vi "Handle pending Requests.vi"(8 "error in (no error)":errorcluster, 11 "IP Connection in":refnum<class "IP Connection.lvclass">) -> (0 "error out":errorcluster, 3 "IP Connection out":refnum<class "IP Connection.lvclass">)   [LabVIEW 2011, in "Tinkerforge.lvlib" / "IP Connection.lvclass"]
doc: "This VI handles pending requests and sends an timeout answer if necessary."
uses:
  IP Connection.lvclass
  IP Connection.lvclass/IP Connection.ctl
  Type Definitions/Request Identifier.ctl
  Type Definitions/Errors.ctl
  Type Definitions/Request Type.ctl
  Type Definitions/Answer.ctl
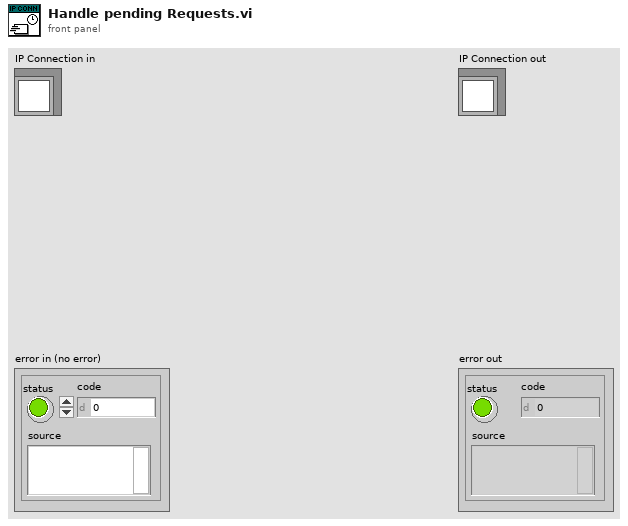
[diagram p1: front panel]
types:
  T1 = typedef "Tinkerforge.lvlib/IP Connection.lvclass/Request Identifier.ctl" = cluster{"Stack ID":u8, "Function ID":u8, "Request GUID":string, "Remaining Timeout":i32}
  T2 = typedef "Tinkerforge.lvlib/IP Connection.lvclass/Errors.ctl" = enum16{"Timeout", "Device type incorrect", "Device already added", "Device not existing"}
  T3 = typedef "Tinkerforge.lvlib/IP Connection.lvclass/Request Type.ctl" = enum8{"Invalid", "Write"}
  T4 = typedef "Tinkerforge.lvlib/IP Connection.lvclass/Answer.ctl" = cluster{"Request GUID":string, "Request Type":T3, "Sucessful":bool, "Data":variant, "Error":errorcluster}
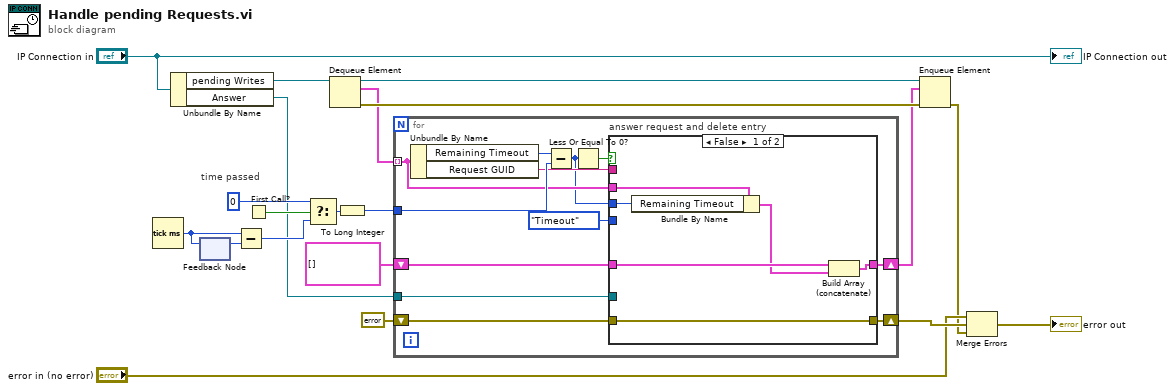
[diagram p0: block diagram]
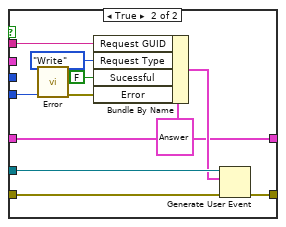
[diagram p2: hidden frame]
diagram:
  # "time passed"
  n1 = Tick Count (ms)() -> (millisecond timer value=w14:u32)
  n2 = Unbundle By Name("IP Connection in") -> ("pending Writes"=w18:refnum<queue>, "Answer"=w7:refnum<user-event>)
  n3 = feedback #1() -> (w15:u32)  [unwired: 1 in]
  n4 = feedback-in #1(w14) -> ()
  n5 = Subtract(x=w14, y=w15) -> (x-y=w13:u32)
  n6 = First Call?() -> (First Call?: T/F=w12:bool)
  n7 = Select(t=u32 0, s=w12, f=w13) -> (s? t:f=w10:u32)
  n8 = Dequeue Element(queue=w18) -> (queue out=w17:refnum<queue>, element=w8:T1[], error out=w16:errorcluster)  [unwired: 2 in, 1 out]
  n9 = To Long Integer(number=w10) -> (32bit integer=w9:i32)
  n10 = for {
    tunnel: w8 -> [w24] mode=indexing
    tunnel: w9 -> [w31]
    shift-right: [w23] -> w5
    shift-left: T1[] [] -> [w28]
    shift-right: [w27] -> w4
    shift-left: errorcluster {"status"=FALSE, "code"=0, "source"=""} ("error out") -> [w30]
    tunnel: w7 -> [w25]
    n11 = Unbundle By Name(w24) -> ("Remaining Timeout"=w32:i32, "Request GUID"=w26:string)
    n12 = Subtract(x=w32, y=w31) -> (x-y=w21:i32)
    n13 = Less Or Equal To 0?(x=w21) -> (x <= 0?=w29:bool)
    n14 = case "answer request and delete entry" shown="False" w29 {
      tunnel: w30 -> [w36 w49]
      tunnel: w28 -> [w38 w41]
      tunnel: [w36 w48] -> w27
      tunnel: w26 -> [_ w44]
      tunnel: w25 -> [_ w43]
      tunnel: w24 -> [w35 _]
      tunnel: [w37 w41] -> w23
      tunnel: Errors."Timeout" ("Error") -> [_ w39]
      tunnel: w21 -> [w33 _]
      frame False {
        n15 = Bundle By Name(cluster=w35, "Remaining Timeout"=w33) -> (w34:T1)
        n16 = Build Array (concatenate)(w38, w34) -> (w37:T1[])
      }
      frame True {
        n17 = call "Error.vi"("Error"=w39) -> ("error cluster"=w40:errorcluster)  [unwired: 10 in]
        n18 = Bundle By Name(cluster=T4 {"Request GUID"="", "Request Type"=enum."Invalid", "Sucessful"=FALSE, "Data"=variant, "Error"={"status"=FALSE, "code"=0, "source"=""}} ("event data"), "Request GUID"=w44, "Request Type"=Request_Type."Write", "Sucessful"=FALSE, "Error"=w40) -> (w42:T4)
        n19 = Generate User Event(user event=w43, event data cluster=w42, error in=w49) -> (error out=w48:errorcluster)  [unwired: 1 out]
      }
    }
  }
  n20 = Enqueue Element(queue=w17, element=w5, error in (no error)=w16) -> (error out=w2:errorcluster)  [unwired: 1 in, 2 out]
  n21 = Merge Errors("error in (no error)", w4, w2) -> (→"error out":errorcluster)
  "IP Connection out" <- "IP Connection in"
